vi "Test Convert.vi"(11 "Error in":errorcluster) -> (15 "Error out":errorcluster)   [LabVIEW 2020, in "CelsiusToFarenheitTests.lvlib"]
doc: "This VI is to validate Celsius to farenheit"
uses:
  CelsiusToFarenheitTests.lvlib
  <vilib>/SLL Drona/APIs/Stimulus/ControlValue/ValueSignalByPathString.vi
  <vilib>/SLL Drona/APIs/Assert/AssertControlValue/AlmostEqual.vi
  <vilib>/SLL Drona/APIs/Stimulus/VI/CloseVI.vi
  <vilib>/SLL Drona/Drona.lvlib
  <vilib>/addons/_JKI Toolkits/Caraya/classes/Test/Test.lvclass
  <vilib>/SLL Drona/APIs/Stimulus/VI/VI.lvlib
  <vilib>/SLL Drona/APIs/Stimulus/ControlValue/ControlValue.lvlib
  <vilib>/SLL Drona/APIs/Assert/AssertControlValue/AssertControlValue.lvlib
panel:
  # "CELSIUS TO FAHRENHEIT TEST"
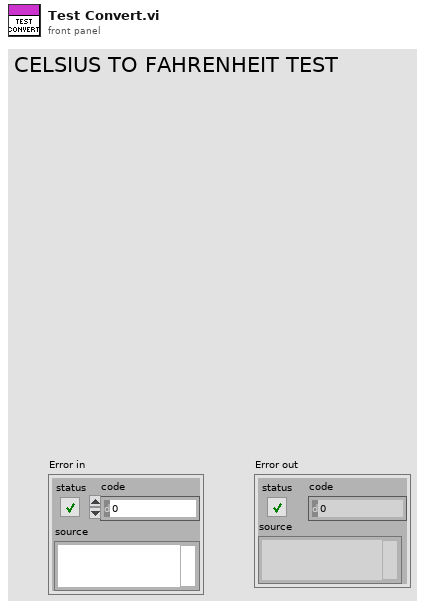
[diagram p1: front panel]
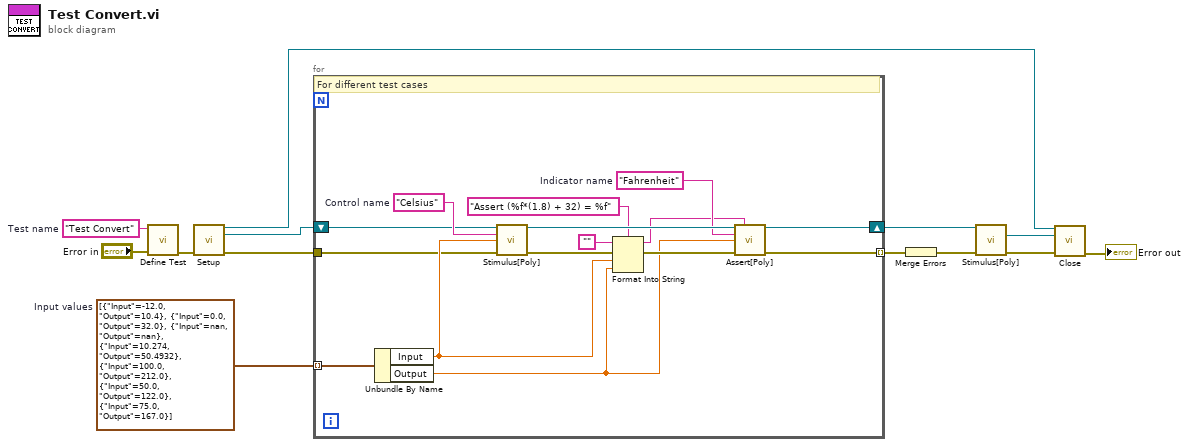
[diagram p0: block diagram]
diagram:
  w4 = "Test Convert"  # Test name
  w12 = cluster{"Input":dbl, "Output":dbl}[] [{"Input"=-12.0, "Output"=10.4}, {"Input"=0.0, "Output"=32.0}, {"Input"=nan, "Output"=nan}, {"Input"=10.274, "Output"=50.4932}, {"Input"=100.0, "Output"=212.0}, {"Input"=50.0, "Output"=122.0}, {"Input"=75.0, "Output"=167.0}]  # Input values
  n1 = call <vilib>:"Define Test.vi"("error in (no error)"="Error in", "Label (VI Title)"=w4) -> ("error out"=w13:errorcluster)  [unwired: 9 in]
  n2 = call <vilib>:"Setup.vi"("error in"=w13) -> ("Application Ref"=w10:refnum<vi>, "VI Reference Out"=w11:refnum<vi>, "error out"=w5:errorcluster)  [unwired: 12 in]
  n3 = for {
    tunnel: w12 -> [w28] mode=indexing
    shift-right: [w18] -> w9
    shift-left: w11 -> [w26]
    tunnel: w5 -> [w15]
    tunnel: [w14] -> w7 mode=indexing
    w19 = "Fahrenheit"  # Indicator name
    w27 = "Celsius"  # Control name
    # "For different test cases"
    n4 = Unbundle By Name(w28) -> ("Input"=w16:dbl, "Output"=w20:dbl)
    n5 = call-poly <vilib>:"Stimulus[Poly].vi"("VI Reference In"=w26, "Control Path"=w27, "Value (Signaling)"=w16, "error in"=w15) -> ("VI Reference Out"=w22:refnum<vi>, "error out"=w24:errorcluster)  [unwired: 10 in]
    n6 = Format Into String(format string="Assert (%f*(1.8) + 32) = %f", initial string="", error in=w24, w16, w20) -> (resulting string=w17:string, error out=w23:errorcluster)
    n7 = call-poly <vilib>:"Assert[Poly].vi"("VI Reference In"=w22, "Test Label"=w17, "Control Path"=w19, "Control Value"=w20, "Error In"=w23) -> ("VI Reference Out"=w18:refnum<vi>, "Error Out"=w14:errorcluster)  [unwired: 9 in]
  }
  n8 = Merge Errors(w7) -> (w2:errorcluster)
  n9 = call-poly <vilib>:"Stimulus[Poly].vi"("VI Reference In"=w9, "error in"=w2) -> ("VI Reference Out"=w8:refnum<vi>, "error out"=w6:errorcluster)  [unwired: 12 in]
  n10 = call <vilib>:"Close.vi"("Application Ref"=w10, "VI Reference"=w8, "error in"=w6) -> ("error out"=→"Error out":errorcluster)  [unwired: 12 in]
